vi "LoadDampValues.vi"(8 "error in (no error)":errorcluster) -> (0 "error out":errorcluster)   [LabVIEW 2015]
uses:
  Drive/Implementation/Damp Type Def.ctl
  <vilib>/Rock Robotics/Network Tables/NT Read Numeric Array.vi
  Drive/Implementation/RobotDriveGlobal.vi
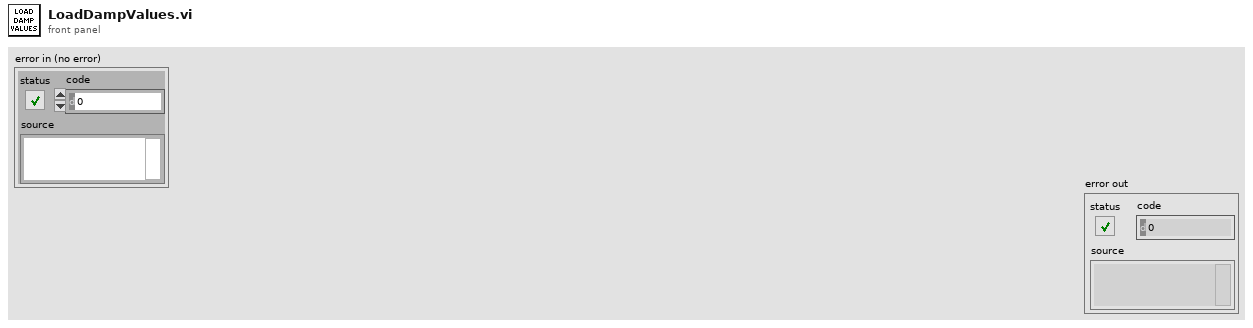
[diagram p1: front panel]
types:
  T1 = typedef "Damp Type Def.ctl" = cluster{"Start Damp":dbl, "Min Speed":dbl}
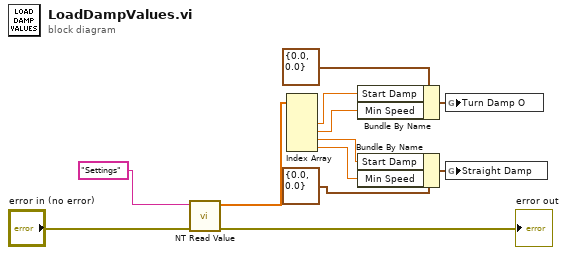
[diagram p0: block diagram]
diagram:
  n1 = call-poly <vilib>:"NT Read Value.vi"("error in"="error in (no error)", "Name"="Settings") -> ("error out"=→"error out":errorcluster, "Numeric Array"=w12:dbl[])  [unwired: 8 in]
  n2 = Index Array(array=w12) -> (element #2=w7:dbl, element #3=w6:dbl, element #4=w5:dbl, element #5=w4:dbl)  [unwired: 5 in, 1 out]
  n3 = Bundle By Name(cluster=T1 {"Start Damp"=0.0, "Min Speed"=0.0} ("Turn Damp"), "Start Damp"=w7, "Min Speed"=w6) -> (w2:T1)
  n4 = Bundle By Name(cluster=T1 {"Start Damp"=0.0, "Min Speed"=0.0} ("Turn Damp"), "Start Damp"=w5, "Min Speed"=w4) -> (w3:T1)
  n5 = global write "RobotDriveGlobal.vi" "Turn Damp O"(w2) -> ()
  n6 = global write "RobotDriveGlobal.vi" "Straight Damp"(w3) -> ()
